vi "PH_SHS_Analysis_Statistician.evt Call Select Data.vi"(0 "i ref in":refnum<vi>, 1 "Stat or Trend":bool, 2 "Data 1":i16, 3 "Data 2":i16, 4 "Data 3":i16, 5 "error in (no error)":errorcluster, 6 "Instance":string="N/A") -> (14 "i ref out":refnum<vi>, 19 "error out":errorcluster)   [LabVIEW 2014, in "PH_SHS_Analysis_Statistician.lvlib"]
doc: "This VI calls a certain ProcCase"
uses:
  PH_SHS_Analysis_Statistician.lvlib
  CS_Core/CSSystem/CoreLib/CoreLib.short 2 byte array.vi
  CS_Core/BaseProcess/BaseProcess.lvlib
  CS_Core/CSSystem/CoreLib/CoreLib.lvlib
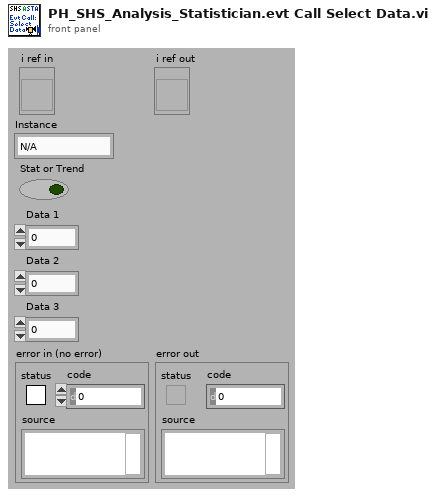
[diagram p1: front panel]
types:
  T1 = typedef "CoreDefs.rawDataType.ctl" = i8[]
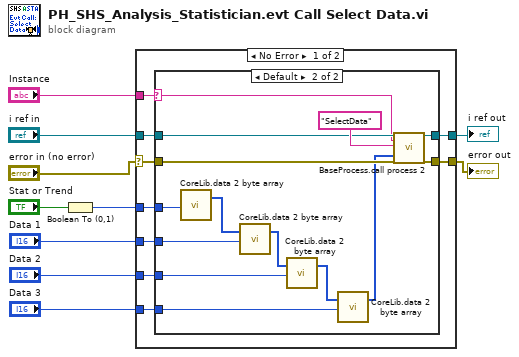
[diagram p0: block diagram]
diagram:
  n1 = Boolean To (0,1)(Boolean="Stat or Trend") -> (0, 1=w4:i16)
  n2 = case shown="No Error" "error in (no error)" {
    selector: "error in (no error)" -> [w15 w36]
    tunnel: [w19 w37] -> w10
    tunnel: [w18 w36] -> w9
    tunnel: "i ref in" -> [w17 w37]
    tunnel: "Instance" -> [w16 _]
    tunnel: w4 -> [w14 _]
    tunnel: "Data 1" -> [w13 _]
    tunnel: "Data 2" -> [w12 _]
    tunnel: "Data 3" -> [w11 _]
    frame No Error {
      n3 = case shown="Default" w16 {
        selector: w16 -> [_ w30]
        tunnel: [w21 w33] -> w19
        tunnel: [w20 w32] -> w18
        tunnel: w17 -> [w21 w31]
        tunnel: w15 -> [w20 w35]
        tunnel: w14 -> [_ w29]
        tunnel: w13 -> [_ w24]
        tunnel: w12 -> [_ w23]
        tunnel: w11 -> [_ w22]
        frame "N/A" {
        }
        frame Default {
          n4 = call-poly "CoreLib.data 2 byte array.vi"("i16"=w29) -> ("byteArray out"=w26:T1)  [unwired: 18 in]
          n5 = call-poly "CoreLib.data 2 byte array.vi"("byteArray"=w26, "i16"=w24) -> ("byteArray out"=w28:T1)  [unwired: 17 in]
          n6 = call-poly "CoreLib.data 2 byte array.vi"("byteArray"=w28, "i16"=w23) -> ("byteArray out"=w27:T1)  [unwired: 17 in]
          n7 = call-poly "CoreLib.data 2 byte array.vi"("byteArray"=w27, "i16"=w22) -> ("byteArray out"=w25:T1)  [unwired: 17 in]
          n8 = call "BaseProcess.call process 2.vi"("i ref in"=w31, "Object"=w30, "Selector"="SelectData", "Data"=w25, "error in (no error)"=w35) -> ("i ref out"=w33:refnum<vi>, "error out"=w32:errorcluster)  [unwired: 13 in]
        }
      }
    }
    frame Error {
    }
  }
  "error out" <- w9
  "i ref out" <- w10
